vi "Pockels Cal-Extract conditions.vi"(11 "Pockels Cal table (full)":string[][](array[string])=[["Cal Wavelength", "", "", ""], ["820", "", "", ""], ["Prism 1:", "2039", "", ""], ["Prism 2:", "1953", "", ""], ["Laser power displayed (mW):", "3960", "", ""], ["Pockels bias:", "199", "", ""], ["Zoom:", "12", "", ""], ["Dwell time:", "0.4", "", ""], ["Cal subset indexes", "", "", ""], ["0", "15", "", ""], ["Cal data", "", "", ""], ["Pockels V", "No objective", "Nikon X", "Nikon 25X"], ["0", "0", "", "0"], ["0.1", "2.8", "", "1.96"], ["0.2", "9.8", "", "6.86"], ["0.3", "21.4", "", "14.98"], ["0.4", "37.1", "", "25.97"], ["0.5", "56.1", "", "39.27"], ["0.6", "77.7", "", "54.39"], ["0.7", "101", "", "70.7"], ["0.8", "125", "", "87.5"], ["0.9", "148", "", "103.6"], ["1", "169", "", "118.3"], ["1.1", "188", "", "131.6"], ["1.2", "204", "", "142.8"], ["1.3", "215", "", "150.5"], ["1.4", "222", "", "155.4"], ["1.5", "225", "", "157.5"], ["1.6", "222", "", "155.4"], ["1.7", "214", "", "149.8"], ["1.8", "202", "", "141.4"], ["1.9", "187", "", "130.9"], ["2", "152", "", "106.4"]]) -> (0 "Required Info Found?":bool, 1 "Pockels cal conditions row index":T1, 3 "Pockels cal conditions":T2)   [LabVIEW 2017]
uses:
  Typedefs/Pockels cal conditions cluster.ctl
  Typedefs/Pockels cal conditions row indexes cluster.ctl
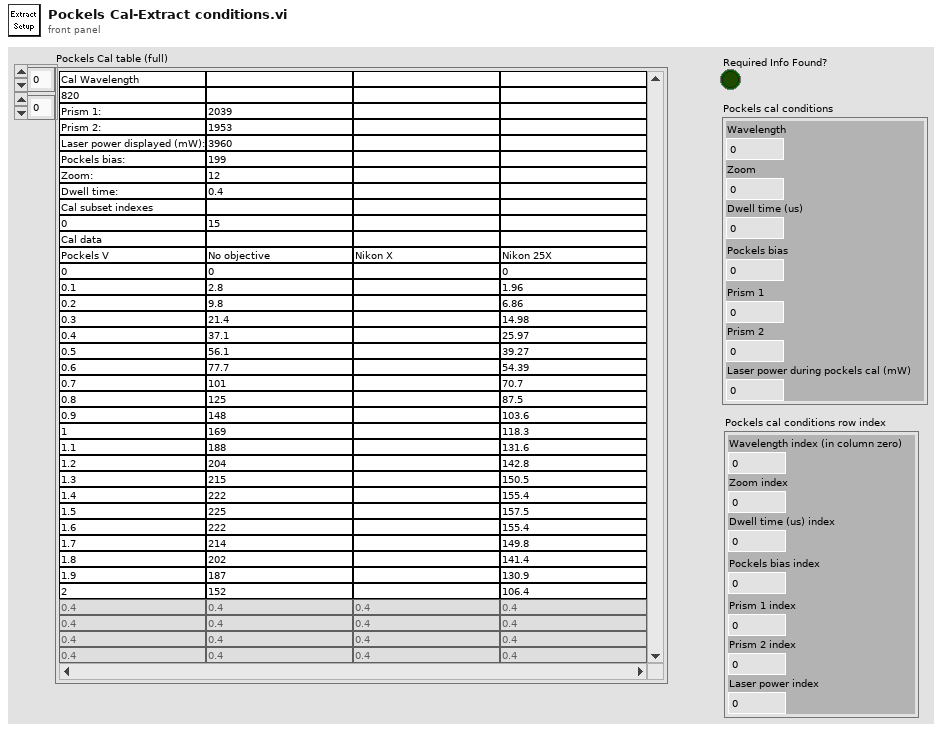
[diagram p1: front panel]
types:
  T1 = typedef "Pockels cal conditions row indexes cluster.ctl" = cluster{"Wavelength index (in column zero)":i32, "Zoom index":i32, "Dwell time (us) index":i32, "Pockels bias index":i32, "Prism 1 index":i32, "Prism 2 index":i32, "Laser power index":i32}
  T2 = typedef "Pockels cal conditions cluster.ctl" = cluster{"Wavelength":u16, "Zoom":u8, "Dwell time (us)":dbl, "Pockels bias":i16, "Prism 1":u16, "Prism 2":u16, "Laser power during pockels cal (mW)":u16}
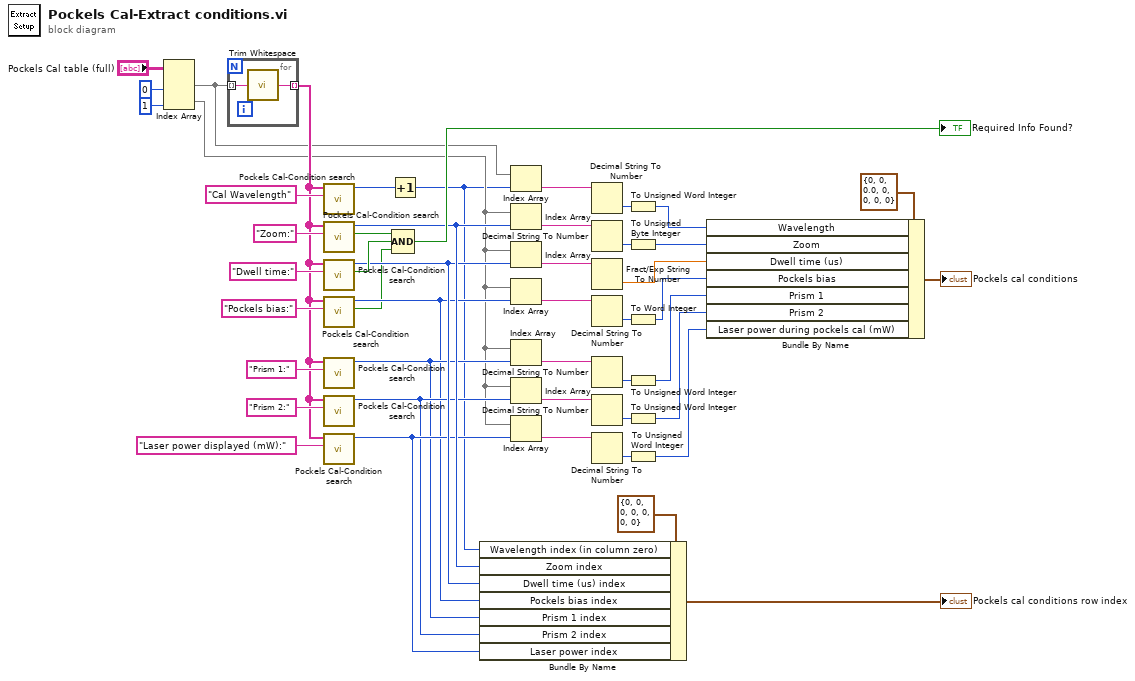
[diagram p0: block diagram]
diagram:
  n1 = Index Array(array="Pockels Cal table (full)", index (col) #1=0 ("disabled index (row)"), index (col) #2=1 ("index (col)")) -> (element #1=w4:string[], element #2=w3:string[])  [unwired: 2 in]
  n2 = for {
    tunnel: w4 -> [w51] mode=indexing
    tunnel: [w50] -> w5 mode=indexing
    n3 = call <vilib>:"Trim Whitespace.vi"("string"=w51) -> ("trimmed string"=w50:string)  [unwired: 1 in]
  }
  n4 = call "Pockels Cal-Condition search.vi"("Condition name"="Cal Wavelength" ("element"), "Pockels Cal table"=w5) -> ("Index"=w9:i32)  [unwired: 8 in, 1 out]
  n5 = call "Pockels Cal-Condition search.vi"("Condition name"="Zoom:" ("element"), "Pockels Cal table"=w5) -> ("Found?"=w45:bool, "Index"=w19:i32)  [unwired: 8 in]
  n6 = call "Pockels Cal-Condition search.vi"("Condition name"="Dwell time:" ("element"), "Pockels Cal table"=w5) -> ("Found?"=w40:bool, "Index"=w18:i32)  [unwired: 8 in]
  n7 = call "Pockels Cal-Condition search.vi"("Condition name"="Pockels bias:" ("element"), "Pockels Cal table"=w5) -> ("Found?"=w10:bool, "Index"=w11:i32)  [unwired: 8 in]
  n8 = call "Pockels Cal-Condition search.vi"("Condition name"="Prism 1:" ("element"), "Pockels Cal table"=w5) -> ("Index"=w12:i32)  [unwired: 8 in, 1 out]
  n9 = call "Pockels Cal-Condition search.vi"("Condition name"="Prism 2:" ("element"), "Pockels Cal table"=w5) -> ("Index"=w13:i32)  [unwired: 8 in, 1 out]
  n10 = call "Pockels Cal-Condition search.vi"("Condition name"="Laser power displayed (mW):" ("element"), "Pockels Cal table"=w5) -> ("Index"=w17:i32)  [unwired: 8 in, 1 out]
  n11 = Increment(x=w9) -> (x+1=w1:i32)
  n12 = Compound Arithmetic op=AND(w45, w40, w10) -> (→"Required Info Found?":bool)
  n13 = Bundle By Name(cluster=T1 {"Wavelength index (in column zero)"=0, "Zoom index"=0, "Dwell time (us) index"=0, "Pockels bias index"=0, "Prism 1 index"=0, "Prism 2 index"=0, "Laser power index"=0} ("Pockels cal conditions row index"), "Wavelength index (in column zero)"=w1, "Zoom index"=w19, "Dwell time (us) index"=w18, "Pockels bias index"=w11, "Prism 1 index"=w12, "Prism 2 index"=w13, "Laser power index"=w17) -> (→"Pockels cal conditions row index":T1)
  n14 = Index Array(array=w4, index=w1) -> (element=w6:string)
  n15 = Index Array(array=w3, index=w19) -> (element=w33:string)
  n16 = Index Array(array=w3, index=w18) -> (element=w39:string)
  n17 = Index Array(array=w3, index=w11) -> (element=w30:string)
  n18 = Index Array(array=w3, index=w12) -> (element=w32:string)
  n19 = Index Array(array=w3, index=w13) -> (element=w31:string)
  n20 = Index Array(array=w3, index=w17) -> (element=w27:string)
  n21 = Decimal String To Number(string=w6) -> (number=w8:i32)  [unwired: 2 in, 1 out]
  n22 = Decimal String To Number(string=w33) -> (number=w42:i32)  [unwired: 2 in, 1 out]
  n23 = Fract/Exp String To Number(string=w39) -> (number=w41:dbl)  [unwired: 3 in, 1 out]
  n24 = Decimal String To Number(string=w30) -> (number=w28:i32)  [unwired: 2 in, 1 out]
  n25 = Decimal String To Number(string=w32) -> (number=w29:i32)  [unwired: 2 in, 1 out]
  n26 = Decimal String To Number(string=w31) -> (number=w24:i32)  [unwired: 2 in, 1 out]
  n27 = Decimal String To Number(string=w27) -> (number=w22:i32)  [unwired: 2 in, 1 out]
  n28 = To Unsigned Word Integer(number=w8) -> (unsigned 16bit integer=w2:u16)
  n29 = To Unsigned Byte Integer(number=w42) -> (unsigned 8bit integer=w20:u8)
  n30 = To Word Integer(number=w28) -> (16bit integer=w14:i16)
  n31 = To Unsigned Word Integer(number=w29) -> (unsigned 16bit integer=w25:u16)
  n32 = To Unsigned Word Integer(number=w24) -> (unsigned 16bit integer=w23:u16)
  n33 = To Unsigned Word Integer(number=w22) -> (unsigned 16bit integer=w21:u16)
  n34 = Bundle By Name(cluster=T2 {"Wavelength"=0, "Zoom"=0, "Dwell time (us)"=0.0, "Pockels bias"=0, "Prism 1"=0, "Prism 2"=0, "Laser power during pockels cal (mW)"=0} ("Setup"), "Wavelength"=w2, "Zoom"=w20, "Dwell time (us)"=w41, "Pockels bias"=w14, "Prism 1"=w25, "Prism 2"=w23, "Laser power during pockels cal (mW)"=w21) -> (→"Pockels cal conditions":T2)
